vi "Power Accuracy Handle Test Complete.vi"(6 "Quick Mode (F)":bool, 8 "error in (no error)":errorcluster, 9 "Test Parameters":T1={"Stimulus"={"Power Start"=38, "Power Stop"=46, "Frequency Type"=enum."Band Edges", "Frequency Points"=[], "TX 1 Frequency (MHz)"={"Min"=0.0, "Max"=0.0}, "TX 2 Frequency (MHz)"={"Min"=0.0, "Max"=0.0}, "RX Frequency (MHz)"={"Min"=0.0, "Max"=0.0}, "Pad Model Number"="", "Pad Serial Number"="", "Pad Values"=[]}, "Measurement"={"DUT Port"=enum."Port 1", "Direction"=0}, "Display"={"Power"={"Min"=-160, "Max"=-60}, "Tolerance"={"Min"=0.0, "Max"=0.0}}, "Limit"={"Tolerance"=0.35}, "Calibration"={"Calibrated?"=FALSE}} {"Measurement"."Direction" items=["Reverse", "Forward", "Auxiliary"]}, 11 "Queue":refnum<queue>) -> (0 "error out":errorcluster)   [LabVIEW 2011]
uses:
  TypeDefs/Power Accuracy Queue Cluster.ctl
  TypeDefs/Power Accuracy Test Parameters.ctl
  TypeDefs/Power Accuracy Stimulus Parameters.ctl
  TypeDefs/Power Accuracy Measurement Parameters.ctl
  SI.LIB/PIM.LIB/HW IO/DUTport.ctl
  SI.LIB/PIM.LIB/HW IO/MeasMode.ctl
  TypeDefs/Power Accuracy Display Parameters.ctl
  TypeDefs/Power Accuracy Limit Parameters.ctl
  TypeDefs/Power Accuracy Calibration State.ctl
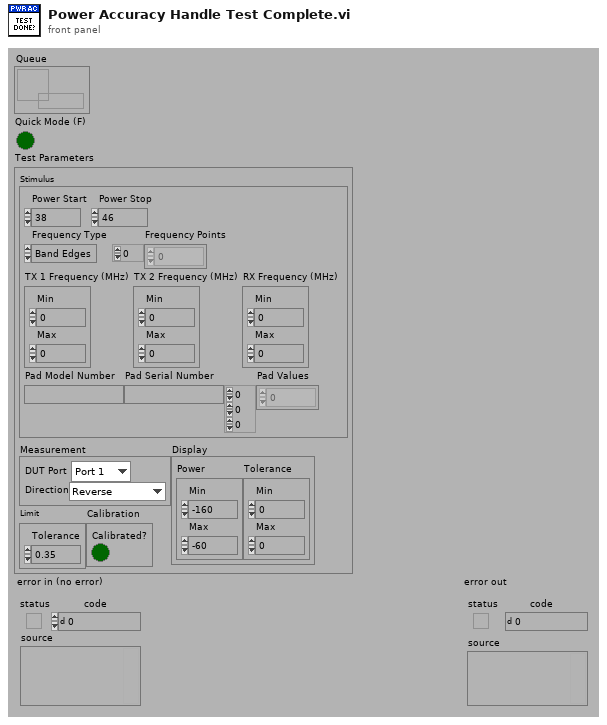
[diagram p1: front panel]
types:
  T1 = typedef "Power Accuracy Test Parameters.ctl" = cluster{"Stimulus":T2, "Measurement":T3, "Display":T6, "Limit":T7, "Calibration":T8}
  T2 = typedef "Power Accuracy Stimulus Parameters.ctl" = cluster{"Power Start":i32, "Power Stop":i32, "Frequency Type":enum16{"Band Edges", "Custom"}, "Frequency Points":dbl[], "TX 1 Frequency (MHz)":cluster{"Min":dbl, "Max":dbl}, "TX 2 Frequency (MHz)":cluster{"Min":dbl, "Max":dbl}, "RX Frequency (MHz)":cluster{"Min":dbl, "Max":dbl}, "Pad Model Number":string, "Pad Serial Number":string, "Pad Values":dbl[][][]}
  T3 = typedef "Power Accuracy Measurement Parameters.ctl" = cluster{"DUT Port":T4, "Direction":T5}
  T4 = typedef "DUTport.ctl" = enum16{"Port 1", "Port 2"}
  T5 = typedef "MeasMode.ctl" = u16
  T6 = typedef "Power Accuracy Display Parameters.ctl" = cluster{"Power":cluster{"Min":i32, "Max":i32}, "Tolerance":cluster{"Min":dbl, "Max":dbl}}
  T7 = typedef "Power Accuracy Limit Parameters.ctl" = cluster{"Tolerance":dbl}
  T8 = typedef "Power Accuracy Calibration State.ctl" = cluster{"Calibrated?":bool}
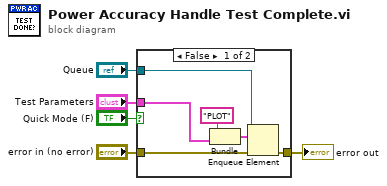
[diagram p0: block diagram]
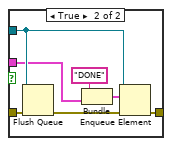
[diagram p2: hidden frame]
diagram:
  n1 = case shown="False" "Quick Mode (F)" {
    tunnel: [w11 w18] -> w5
    tunnel: "Queue" -> [w8 w14]
    tunnel: "error in (no error)" -> [w6 w15]
    tunnel: "Test Parameters" -> [w7 w12]
    frame False {
      n2 = Bundle("PLOT", "Test Parameters"=w7) -> (w9:cluster{string, "Test Parameters":T1})  [unwired: 1 out]
      n3 = Enqueue Element(queue=w8, element=w9, error in (no error)=w6) -> (error out=w11:errorcluster)  [unwired: 3 out]
    }
    frame True {
      n4 = Flush Queue(queue=w14, error in (no error)=w15) -> (error out=w13:errorcluster)  [unwired: 2 out]
      n5 = Bundle("DONE", "Test Parameters"=w12) -> (w16:cluster{string, "Test Parameters":T1})  [unwired: 1 out]
      n6 = Enqueue Element(queue=w14, element=w16, error in (no error)=w13) -> (error out=w18:errorcluster)  [unwired: 3 out]
    }
  }
  "error out" <- w5
